vi "create.AddOrderLong.vi"(8 "error in":errorcluster, 10 "AddOrderLong.Parameters":T1, 11 "AddOrderLong in":refnum<class "AddOrderLong.lvclass">) -> (0 "error out":errorcluster, 3 "AddOrderLong out":refnum<class "AddOrderLong.lvclass">)   [LabVIEW 2022 SP3, in "AddOrderLong.lvclass"]
uses:
  AddOrderLong.lvclass
  AddOrderLong.Parameters.ctl
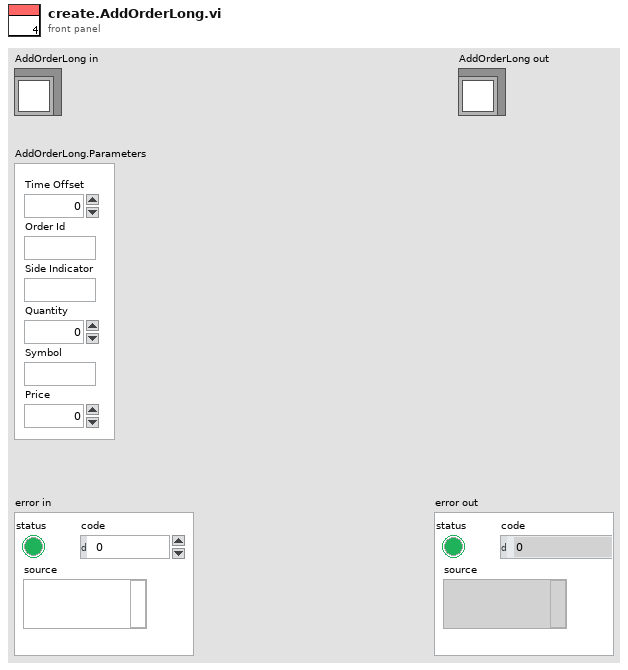
[diagram p1: front panel]
types:
  T1 = typedef "AddOrderLong.lvclass/AddOrderLong.Parameters.ctl" = cluster{"Time Offset":u32, "Order Id":string, "Quantity":u32, "Symbol":string, "Side Indicator":string, "Price":dbl}
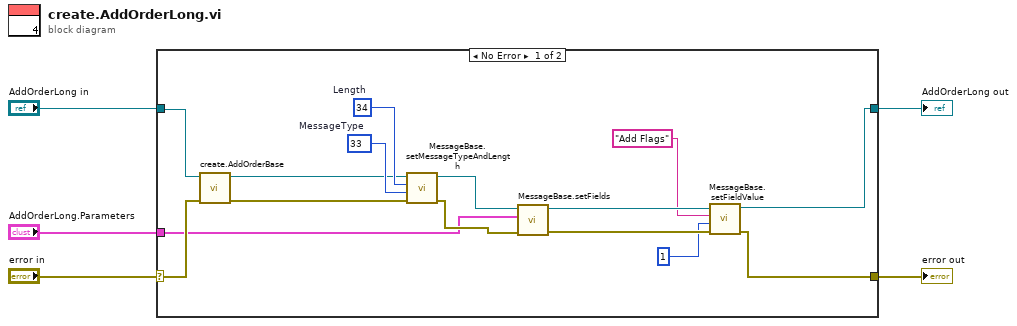
[diagram p0: block diagram]
diagram:
  n1 = case shown="No Error" "error in" {
    selector: "error in" -> [w13 w22]
    tunnel: [w7 w22] -> w4
    tunnel: [w6 w21] -> w2
    tunnel: "AddOrderLong in" -> [w14 w21]
    tunnel: "AddOrderLong.Parameters" -> [w12 _]
    frame No Error {
      w19 = u8 33  # MessageType
      w20 = u8 34  # Length
      n2 = call-dynamic "create.AddOrderBase.vi"("error in (no error)"=w13, "AddOrderBase in"=w14) -> ("error out"=w18:errorcluster, "AddOrderBase out"=w17:refnum<class "AddOrderLong.lvclass">)  [unwired: 8 in]
      n3 = call-dynamic "MessageBase.setMessageTypeAndLength.vi"("error in (no error)"=w18, "MessageType"=w19, "Length"=w20, "MessageBase in"=w17) -> ("error out"=w15:errorcluster, "MessageBase out"=w16:refnum<class "AddOrderLong.lvclass">)  [unwired: 6 in]
      n4 = call-dynamic "MessageBase.setFields.vi"("error in (no error)"=w15, "Cluster (dup)"=w12, "MessageBase in"=w16) -> ("error out"=w10:errorcluster, "MessageBase out"=w11:refnum<class "AddOrderLong.lvclass">)  [unwired: 7 in]
      n5 = call-dynamic "MessageBase.setFieldValue.vi"("error in (no error)"=w10, "Value"=u8 1, "FIeld.Name"="Add Flags", "MessageBase in"=w11) -> ("error out"=w7:errorcluster, "MessageBase out"=w6:refnum<class "AddOrderLong.lvclass">)  [unwired: 6 in]
    }
    frame Error {
    }
  }
  "error out" <- w4
  "AddOrderLong out" <- w2
